vi "test_CCDSetAndGetNumberOfAvgs.vi"(7 "Test should pass":bool=TRUE, 8 "error in":errorcluster, 9 "tear down connection":bool=TRUE, 10 "set-up a connection":bool=TRUE, 11 "device selection":enum16{"monochromator", "CCD", "SCD"}(ring)=enum."CCD") -> (0 "error out":errorcluster)   [LabVIEW 2023]
uses:
  <vilib>/addons/_JKI Toolkits/Caraya/classes/Assert/Assert Equal Value and Type_Variant.vi
  <vilib>/addons/_JKI Toolkits/Caraya/classes/Assert/Assert Not Error.vi
  Classes/GenericDevice/GenericDevice.lvclass
  <vilib>/addons/_JKI Toolkits/Caraya/classes/Test/Test.lvclass
  <vilib>/addons/_JKI Toolkits/Caraya/classes/Assert/Assert.lvclass
  Classes/CCD/CCD.lvclass
  C:/Projects/Horiba/horiba-labview-sdk/Source/Classes/GenericDevice/GenericDevice.lvclass
  C:/Projects/Horiba/horiba-labview-sdk/Source/Classes/CCD/CCD.lvclass
panel:
  # "Connector Pane"
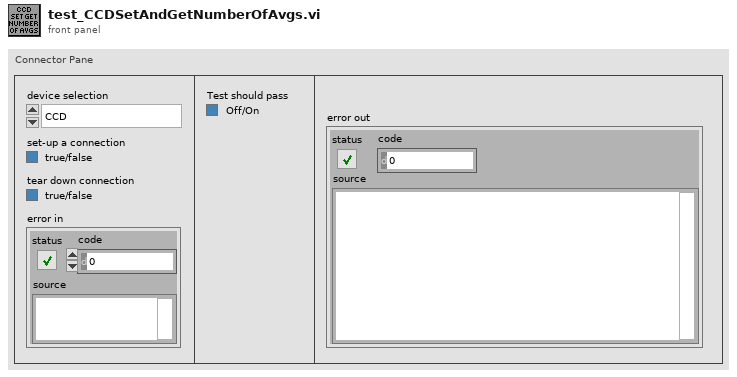
[diagram p1: front panel]
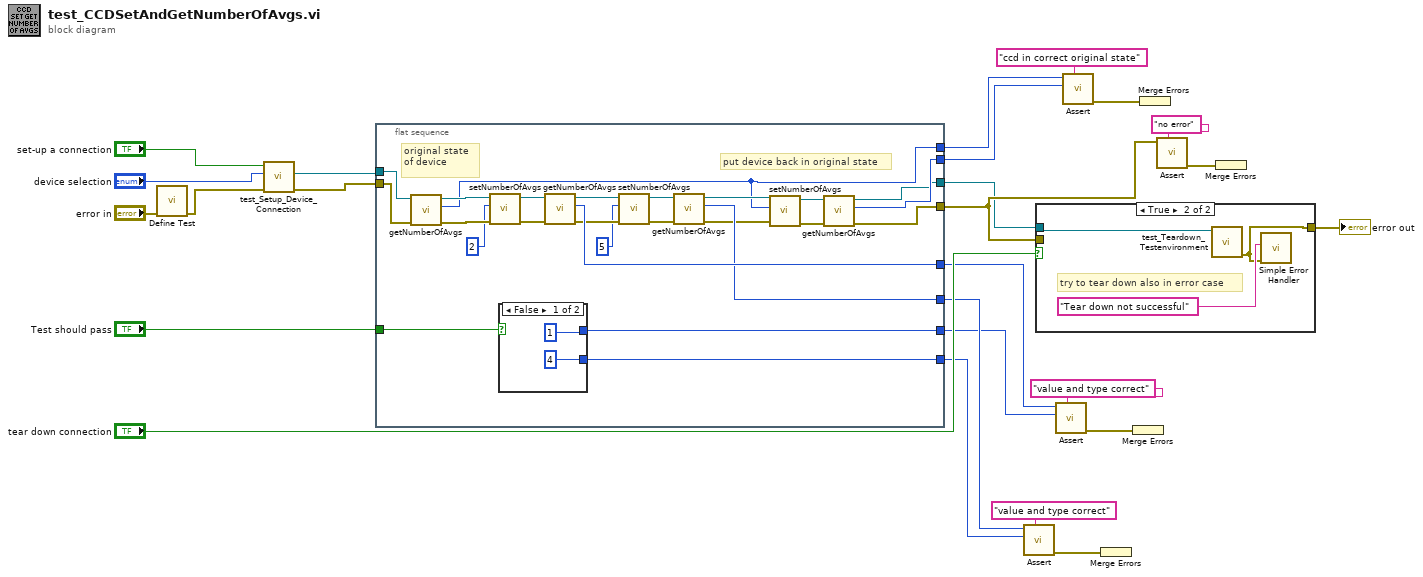
[diagram p0: block diagram]
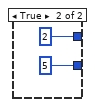
[diagram p2: hidden frame]
diagram:
  n1 = call <vilib>:"Define Test.vi"("error in (no error)"="error in") -> ("error out"=w3:errorcluster)  [unwired: 9 in, 1 out]
  n2 = call "test_Setup_Device_Connection.vi"("error in (no error)"=w3, "device selection"="device selection", "set-up a connection"="set-up a connection") -> ("error out"=w2:errorcluster, "CCD out"=w1:refnum<class "CCD.lvclass">)  [unwired: 5 in, 2 out]
  n3 = flat-sequence {
    tunnel: w2 -> [w46]
    tunnel: w1 -> [w47]
    tunnel: [w26] -> w16
    tunnel: "Test should pass" -> [w50]
    tunnel: [w27] -> w15
    tunnel: [w34] -> w14
    tunnel: [w49] -> w13
    tunnel: [w40] -> w12
    tunnel: [w48] -> w11
    tunnel: [w29] -> w8
    tunnel: [w28] -> w7
    frame #0 {
      # "put device back in original state"
      # "original state of device"
      n4 = call "getNumberOfAvgs.vi"("error in (no error)"=w46, "CCD in"=w47) -> ("error out"=w44:errorcluster, "averages"=w29:i32, "CCD out"=w45:refnum<class "CCD.lvclass">)  [unwired: 7 in]
      n5 = call "setNumberOfAvgs.vi"("error in (no error)"=w44, "number of averages"=2 ("exposure time [ms]"), "CCD in"=w45) -> ("error out"=w42:errorcluster, "CCD out"=w41:refnum<class "CCD.lvclass">)  [unwired: 5 in, 2 out]
      n6 = case shown="False" w50 {
        tunnel: [4 ("exposure time [ms]") 5 ("exposure time [ms]")] -> w49
        tunnel: [1 ("exposure time [ms]") 2 ("exposure time [ms]")] -> w48
        frame False {
        }
        frame True {
        }
      }
      n7 = call "getNumberOfAvgs.vi"("error in (no error)"=w42, "CCD in"=w41) -> ("error out"=w36:errorcluster, "averages"=w40:i32, "CCD out"=w37:refnum<class "CCD.lvclass">)  [unwired: 7 in]
      n8 = call "setNumberOfAvgs.vi"("error in (no error)"=w36, "number of averages"=5 ("exposure time [ms]"), "CCD in"=w37) -> ("error out"=w39:errorcluster, "CCD out"=w38:refnum<class "CCD.lvclass">)  [unwired: 5 in, 2 out]
      n9 = call "getNumberOfAvgs.vi"("error in (no error)"=w39, "CCD in"=w38) -> ("error out"=w31:errorcluster, "averages"=w34:i32, "CCD out"=w32:refnum<class "CCD.lvclass">)  [unwired: 7 in]
      n10 = call "setNumberOfAvgs.vi"("error in (no error)"=w31, "number of averages"=w29, "CCD in"=w32) -> ("error out"=w33:errorcluster, "CCD out"=w30:refnum<class "CCD.lvclass">)  [unwired: 5 in, 2 out]
      n11 = call "getNumberOfAvgs.vi"("error in (no error)"=w33, "CCD in"=w30) -> ("error out"=w26:errorcluster, "averages"=w28:i32, "CCD out"=w27:refnum<class "CCD.lvclass">)  [unwired: 7 in]
    }
  }
  n12 = call-poly <vilib>:"Assert.vi"("Label"="value and type correct" ("Label (VI Title)"), "Y"=w13, "X"=w14) -> ("error out"=w24:errorcluster)  [unwired: 7 in, 1 out]
  n13 = case shown="True" "tear down connection" {
    tunnel: w15 -> [_ w57]
    tunnel: [w55 w56] -> w6
    tunnel: w16 -> [w55 _]
    frame False {
    }
    frame True {
      # "try to tear down also in error case"
      n14 = call "test_Teardown_Testenvironment.vi"("GenericDevice.lvclass"=w57) -> ("error out"=w56:errorcluster)  [unwired: 9 in, 1 out]
      n15 = call <vilib>:"Simple Error Handler.vi"("error source (\" \")"="Tear down not successful" ("error source (\" \")"), "error in (no error)"=w56) -> ()  [unwired: 3 in, 5 out]
    }
  }
  "error out" <- w6
  n16 = call-poly <vilib>:"Assert.vi"("Label"="value and type correct" ("Label (VI Title)"), "Y"=w11, "X"=w12) -> ("error out"=w23:errorcluster)  [unwired: 7 in, 1 out]
  n17 = call-poly <vilib>:"Assert.vi"("Label"="ccd in correct original state" ("Label (VI Title)"), "Y"=w7, "X"=w8) -> ("error out"=w10:errorcluster)  [unwired: 7 in, 1 out]
  n18 = Merge Errors(w24) -> ()  [unwired: 1 out]
  n19 = Merge Errors(w23) -> ()  [unwired: 1 out]
  n20 = Merge Errors(w10) -> ()  [unwired: 1 out]
  n21 = call-poly <vilib>:"Assert.vi"("Label"="no error" ("Label (VI Title)"), "Not Error?"=w16) -> ("error out"=w18:errorcluster)  [unwired: 8 in, 1 out]
  n22 = Merge Errors(w18) -> ()  [unwired: 1 out]
